vi "niFpga wdp fft 4-wire wrapper 8spc.vi"(0 "real data in":fxp<+/-,8,1>[](array[numeric])=[0.0, 0.0, 0.0, 0.0, 0.0, 0.0, 0.0, 0.0], 1 "reset":bool, 5 "imaginary data in":fxp<+/-,8,1>[](array[numeric])=[0.0, 0.0, 0.0, 0.0, 0.0, 0.0, 0.0, 0.0], 9 "input valid":bool, 12 "ready for output":bool) -> (3 "data indices":u16[](array[numeric]), 4 "real data out":fxp<+/-,19,12>[](array[numeric]), 6 "imaginary data out":fxp<+/-,19,12>[](array[numeric]), 10 "output valid":bool, 14 "ready for input":bool)   [LabVIEW 2017]
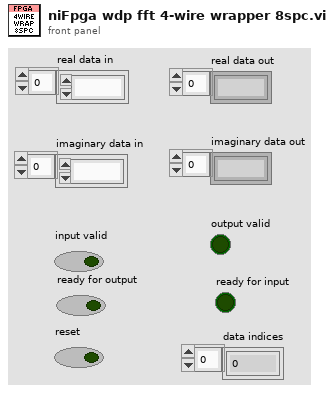
[diagram p1: front panel]
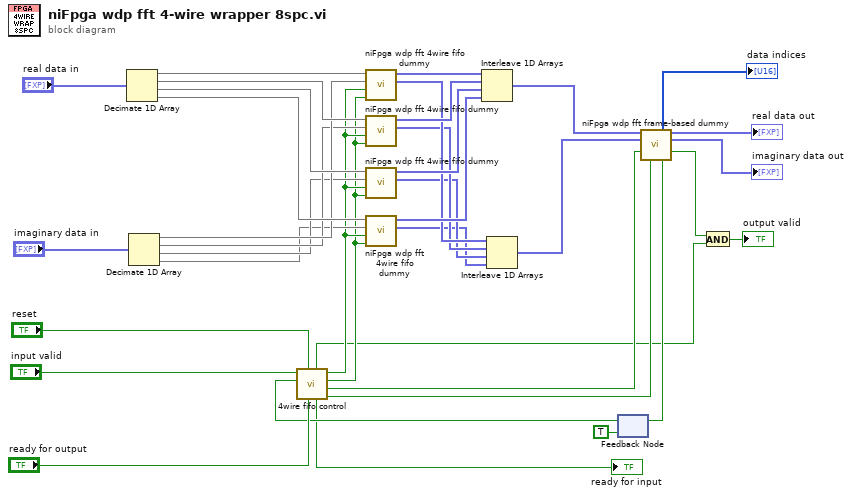
[diagram p0: block diagram]
diagram:
  n1 = Decimate 1D Array("real data in") -> (w29:fxp<+/-,8,1>[], w27:fxp<+/-,8,1>[], w26:fxp<+/-,8,1>[], w25:fxp<+/-,8,1>[])
  n2 = Decimate 1D Array("imaginary data in") -> (w24:fxp<+/-,8,1>[], w23:fxp<+/-,8,1>[], w22:fxp<+/-,8,1>[], w21:fxp<+/-,8,1>[])
  n3 = feedback #1(TRUE ("ready for frame")) -> (w2:bool)
  n4 = call "4wire fifo control"("ready for output"="ready for output", "reset"="reset", "ready for frame"=w2, "input valid"="input valid") -> ("enable"=w10:bool, "frame start"=w9:bool, "read?"=w7:bool, "write?"=w8:bool, "ready for input"=→"ready for input":bool, "not in reset?"=w6:bool)  [unwired: 2 in]
  n5 = call <vilib>:"niFpga wdp fft 4wire fifo dummy.vi"("read?"=w7, "write?"=w8, "data in im"=w24, "data in re"=w29) -> ("data out im"=w16:fxp<+/-,8,1>[], "data out re"=w20:fxp<+/-,8,1>[])  [unwired: 6 in]
  n6 = call <vilib>:"niFpga wdp fft 4wire fifo dummy.vi"("read?"=w7, "write?"=w8, "data in im"=w23, "data in re"=w27) -> ("data out im"=w15:fxp<+/-,8,1>[], "data out re"=w19:fxp<+/-,8,1>[])  [unwired: 6 in]
  n7 = call <vilib>:"niFpga wdp fft 4wire fifo dummy.vi"("read?"=w7, "write?"=w8, "data in im"=w22, "data in re"=w26) -> ("data out im"=w14:fxp<+/-,8,1>[], "data out re"=w18:fxp<+/-,8,1>[])  [unwired: 6 in]
  n8 = call <vilib>:"niFpga wdp fft 4wire fifo dummy.vi"("read?"=w7, "write?"=w8, "data in im"=w21, "data in re"=w25) -> ("data out im"=w13:fxp<+/-,8,1>[], "data out re"=w17:fxp<+/-,8,1>[])  [unwired: 6 in]
  n9 = Interleave 1D Arrays(w20, w19, w18, w17) -> (w12:fxp<+/-,8,1>[])
  n10 = Interleave 1D Arrays(w16, w15, w14, w13) -> (w11:fxp<+/-,8,1>[])
  n11 = call <vilib>:"niFpga wdp fft frame-based dummy.vi"("real data in"=w12, "imaginary data in"=w11, "input frame start"=w9, "enable"=w10) -> ("data indices"=→"data indices":u16[], "real data out"=→"real data out":fxp<+/-,19,12>[], "imaginary data out"=→"imaginary data out":fxp<+/-,19,12>[], "output valid"=w32:bool, "ready for frame"=w33:bool)  [unwired: 6 in, 1 out]
  n12 = feedback-in #1(w33) -> ()
  n13 = And(x=w32, y=w6) -> (x .and. y?=→"output valid":bool)
